vi "GotoFGV.vi"(10 "goto?":bool=TRUE, 11 "goto pos":enum16{"get", "set"}(ring)) -> (3 "moving to position":bool)   [LabVIEW 2020]
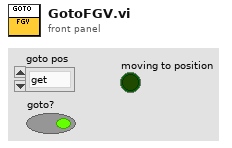
[diagram p1: front panel]
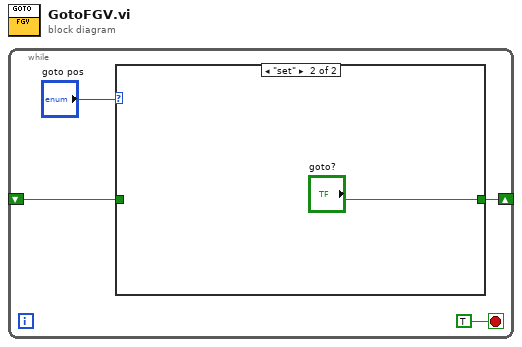
[diagram p0: block diagram]
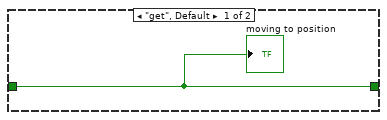
[diagram p2: hidden frame]
diagram:
  n1 = while {
    shift-right: [w3] -> _
    shift-left: _ -> [w2]
    stop <- TRUE stop-if-true
    n2 = case shown="\"set\"" "goto pos" {
      tunnel: [w5 "goto?"] -> w3
      tunnel: w2 -> [w5 _]
      frame "get", Default {
        "moving to position" <- w5
      }
      frame "set" {
      }
    }
  }
